vi "Initialize Theme.vi"(8 "error in (no error)":errorcluster, 11 "Filled Text Fields Actor in":refnum<class "Filled Text Fields Actor.lvclass">) -> (0 "error out":errorcluster, 3 "Filled Text Fields Actor out":refnum<class "Filled Text Fields Actor.lvclass">)   [LabVIEW 2017, in "Filled Text Fields.lvlib" / "Filled Text Fields Actor.lvclass"]
uses:
  Filled Text Fields Actor.lvclass
  Filled Text Fields Actor.lvclass/Filled Text Fields Actor.ctl
  Theme/Theme/Theme.lvclass
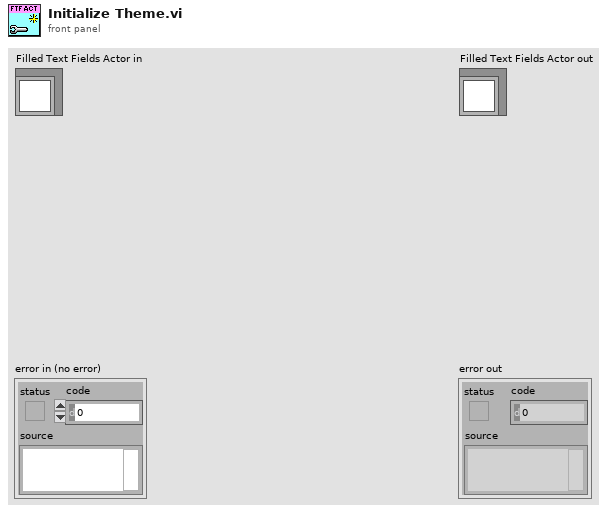
[diagram p1: front panel]
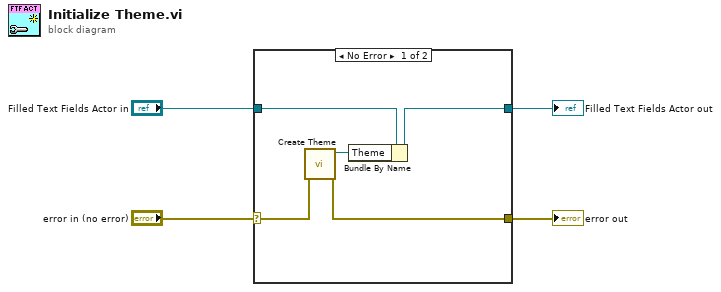
[diagram p0: block diagram]
diagram:
  n1 = case shown="No Error" "error in (no error)" {
    selector: "error in (no error)" -> [w6 w11]
    tunnel: [w5 w11] -> w3
    tunnel: [w8 w10] -> w1
    tunnel: "Filled Text Fields Actor in" -> [w9 w10]
    frame No Error {
      n2 = call "Create Theme.vi"("error in (no error)"=w6) -> ("error out"=w5:errorcluster, "Theme out"=w7:refnum<class "Theme.lvclass">)  [unwired: 9 in]
      n3 = Bundle By Name(cluster=w9, "Theme"=w7) -> (w8:refnum<class "Filled Text Fields Actor.lvclass">)
    }
    frame Error {
    }
  }
  "error out" <- w3
  "Filled Text Fields Actor out" <- w1
